vi "execute.vi"(8 "error in (no error)":errorcluster, 10 "Context in":refnum<class "Context.lvclass">, 11 "RaiseM1M3Command in":refnum<class "RaiseM1M3Command.lvclass">) -> (0 "error out":errorcluster, 2 "Context out":refnum<class "Context.lvclass">, 3 "RaiseM1M3Command out":refnum<class "RaiseM1M3Command.lvclass">)   [LabVIEW 2016, in "RaiseM1M3Command.lvclass"]
uses:
  RaiseM1M3Command.lvclass
  Context/Context.lvclass
  RaiseM1M3Command.lvclass/RaiseM1M3Command.ctl
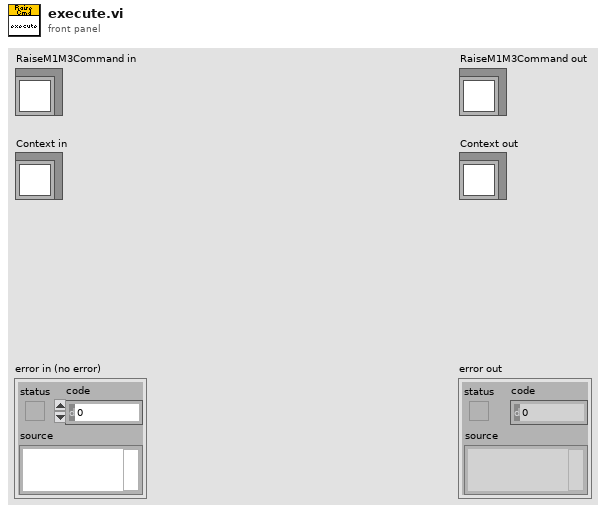
[diagram p1: front panel]
types:
  T1 = typedef "M1M3SupportTopics.lvlib/CommandRaiseM1M3.ctl" = cluster{"CommandId":T2, "RaiseM1M3":bool}
  T2 = typedef "M1M3SupportTopics.lvlib/CommandId.ctl" = i32
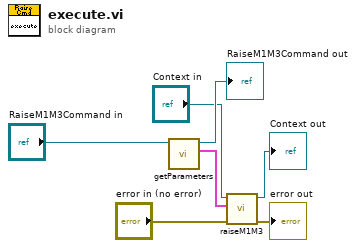
[diagram p0: block diagram]
diagram:
  n1 = call "getParameters.vi"("RaiseM1M3Command in"="RaiseM1M3Command in") -> ("Parameters"=w5:T1, "RaiseM1M3Command out"=→"RaiseM1M3Command out":refnum<class "RaiseM1M3Command.lvclass">)  [unwired: 9 in]
  n2 = call-dynamic "raiseM1M3.vi"("error in (no error)"="error in (no error)", "Parameters"=w5, "Context in"="Context in") -> ("error out"=→"error out":errorcluster, "Context out"=→"Context out":refnum<class "Context.lvclass">)  [unwired: 7 in]
